vi "MAIN - Car Wash.vi"() -> ()   [LabVIEW 2015, in "Car Wash.lvlib"]
uses:
  Car Wash.lvlib
  Components/State Declaration.ctl
  Components/System Trigger.ctl
  Components/System Trigger Element.ctl
  <vilib>/Utility/error.llb/DialogTypeEnum.ctl
  Components/AMC/Read Termination Message.vi
  Components/AMC/Update Message Routing Info.vi
  Components/AMC/Create Multiple Messages.vi
  Components/AMC/Create Single Message.vi
  Components/AMC/Globals.vi
  Components/AMC/Send Message.vi
  Components/TypeDef - SHIFTER.ctl
  Components/Dependencies.llb/TLB`_Dependencies.lvlib
  Components/AMC/AMC.lvlib
panel:
  out "Status":string
  in  "Start Wash":bool
  in  "Reset Car":bool
  out "Wash Progress":i32(slide) scale=0.0..6.0
  in  "Giant Blowdryers":bool
  in  "Rinse":bool
  in  "Wax":bool
  in  "Roller Brushes":bool
  in  "Soap":bool
  in  "Pre-Soak":bool
  out "error out":errorcluster
  # "Car Wash"
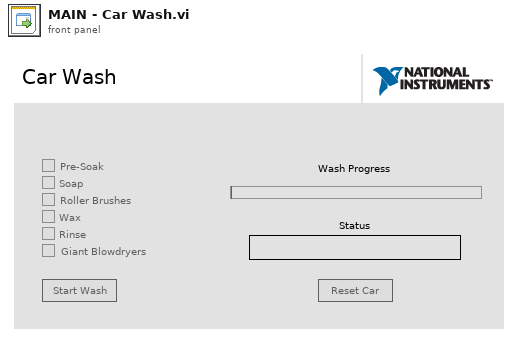
[diagram p1: front panel]
types:
  T1 = typedef "Car Wash.lvlib/System Trigger.ctl" = enum16{"<None>", "Cache User Parameters", "Close Application", "Start Wash", "Reset Car"}
  T2 = typedef "Car Wash.lvlib/State Declaration.ctl" = enum16{"<Startup>", "Idle", "Washing", "<Shutdown>"}
  T3 = enum16{"Clear SR", "Set Display", "Set Shifter", "Initialize Events", "Init Q"}
  T4 = typedef "Car Wash.lvlib/TypeDef - SHIFTER.ctl" = cluster{"State":T2, "User Data":cluster{"Active Item Tag":string, "Pre-Soak":bool, "Soap":bool, "Roller Brushes":bool, "Wax":bool, "Rinse":bool, "Giant Blowdryers":bool}, "Display Data":cluster{"Active Item Tag":string, "Wash Progress":i32, "Status":string}, "User Parameter Controls":refnum<vi>[], "Framework Data":cluster{"Exit Event":T5, "Terminate Error":errorcluster}, "Private Data":cluster{"Active Item Tag":string, "Step Booleans Array":bool[], "Step Names Array":string[], "Wash Done?":bool, "Step Duration":i32}}
  T5 = typedef "Car Wash.lvlib/TLB`_Dependencies.lvlib/Exit Event Ref.ctl" = refnum<user-event>
  T6 = typedef "Car Wash.lvlib/System Trigger Element.ctl" = cluster{"System Triggers":T1, "Trigger Data":variant}
  T7 = typedef "Car Wash.lvlib/AMC.lvlib/Message Queue.ctl" = refnum<queue>
  T8 = enum8{"Enabled", "Disabled", "Disabled and Grayed Out"}
  T9 = typedef "DialogTypeEnum.ctl" = enum16{"no dialog", "OK message", "continue or stop message", "auto error handling dialog", "OK message + warnings", "continue/stop + warnings"}
  T10 = enum32{"Invalid", "Standard", "Closed", "Hidden", "Minimized", "Maximized"}
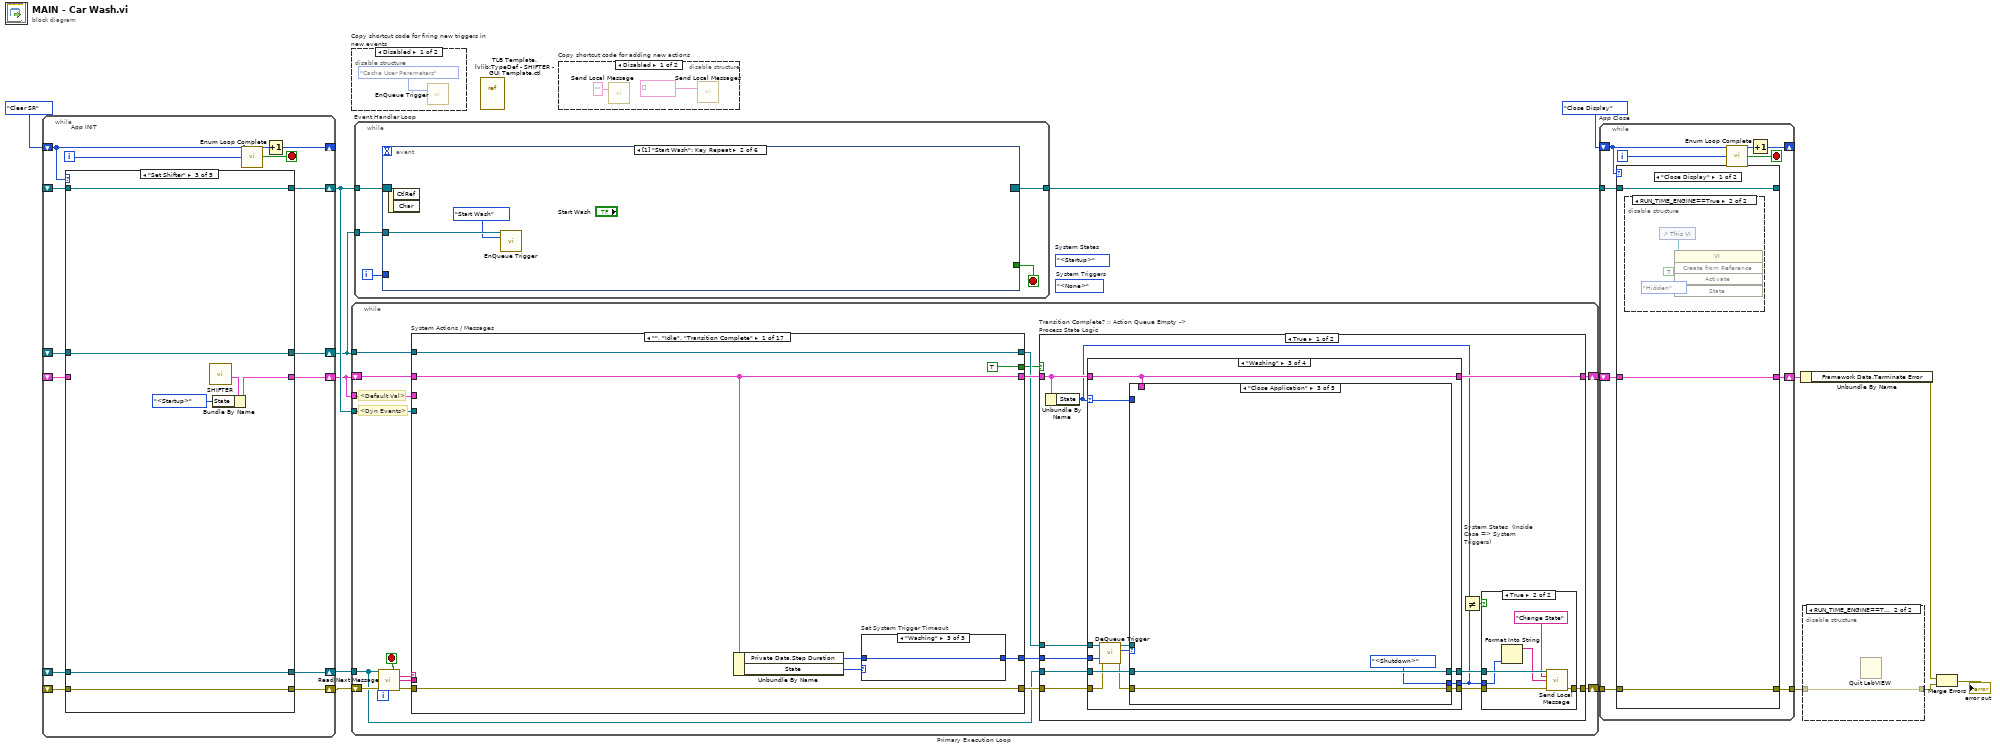
[diagram p0: block diagram]
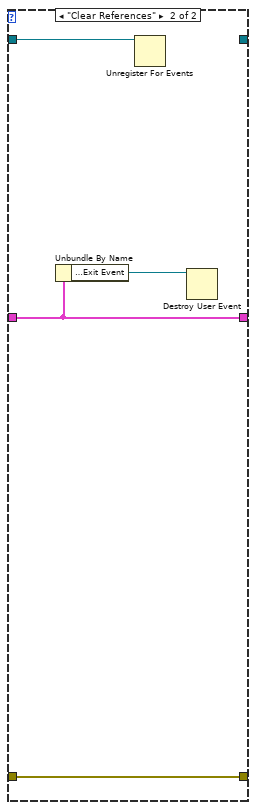
[diagram p6: hidden frame]
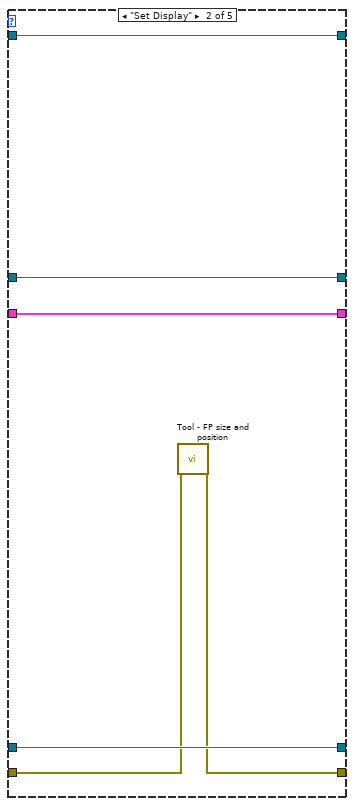
[diagram p8: hidden frame]
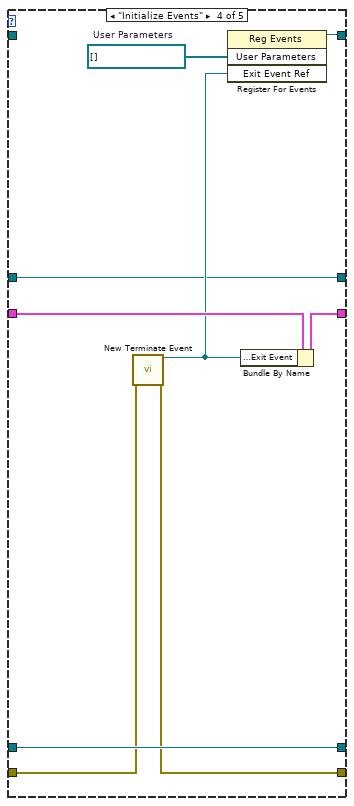
[diagram p9: hidden frame]
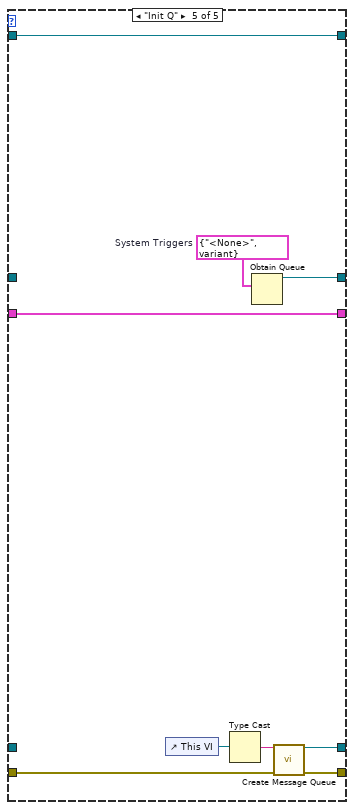
[diagram p10: hidden frame]
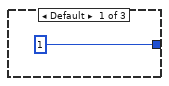
[diagram p11: hidden frame]
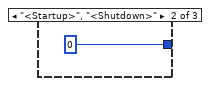
[diagram p12: hidden frame]
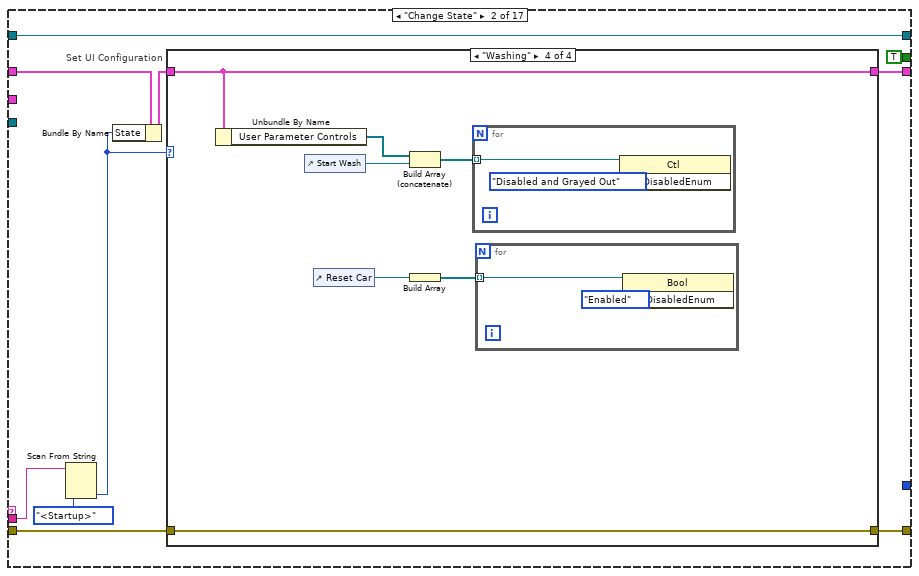
[diagram p13: hidden frame]
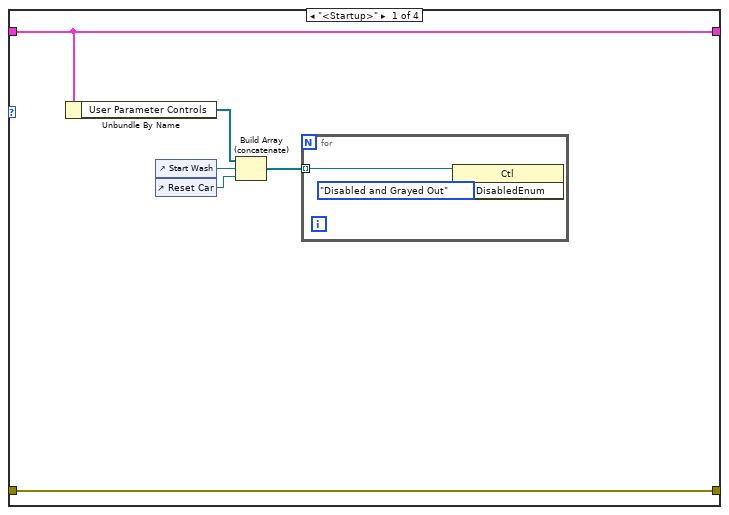
[diagram p14: hidden frame]
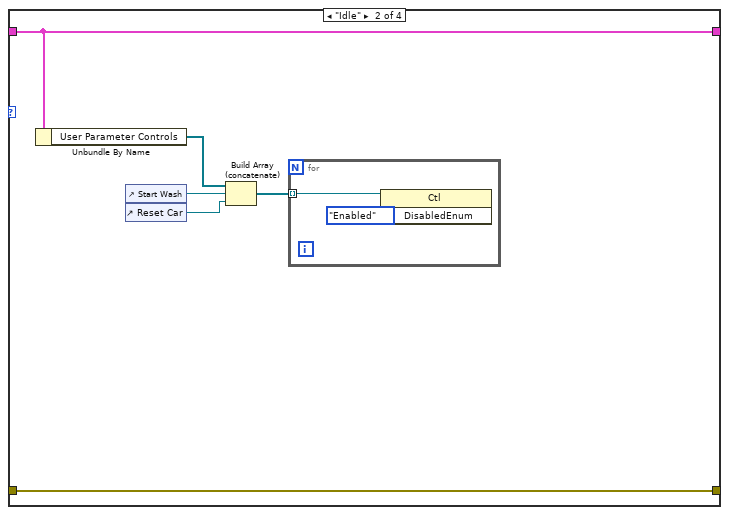
[diagram p15: hidden frame]
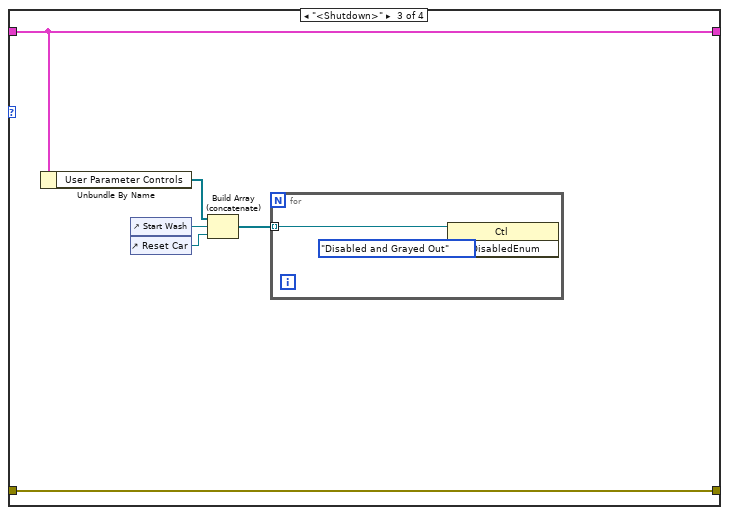
[diagram p16: hidden frame]
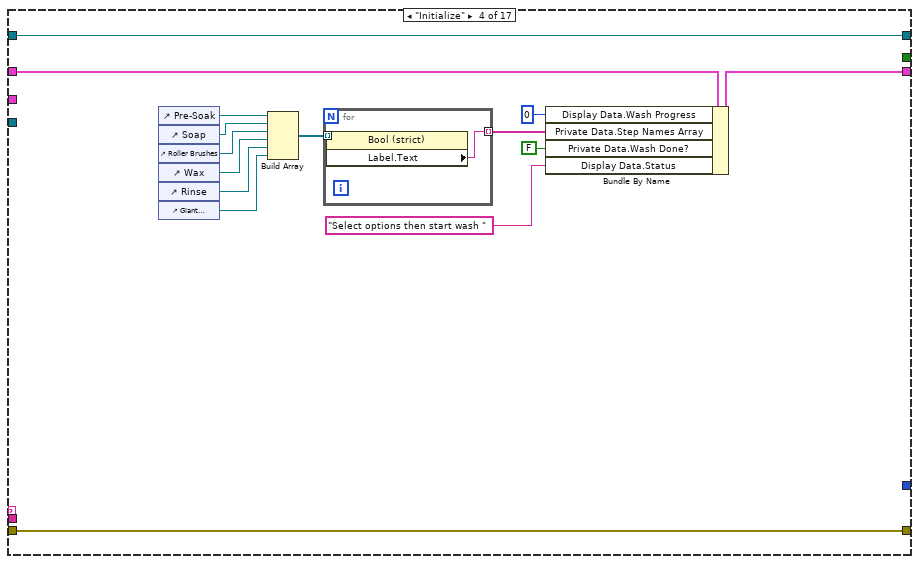
[diagram p18: hidden frame]
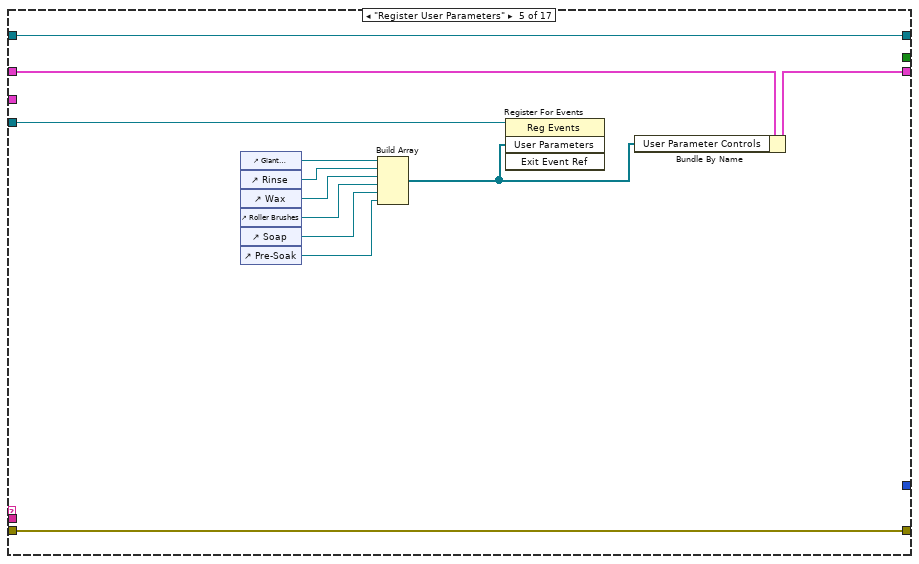
[diagram p19: hidden frame]
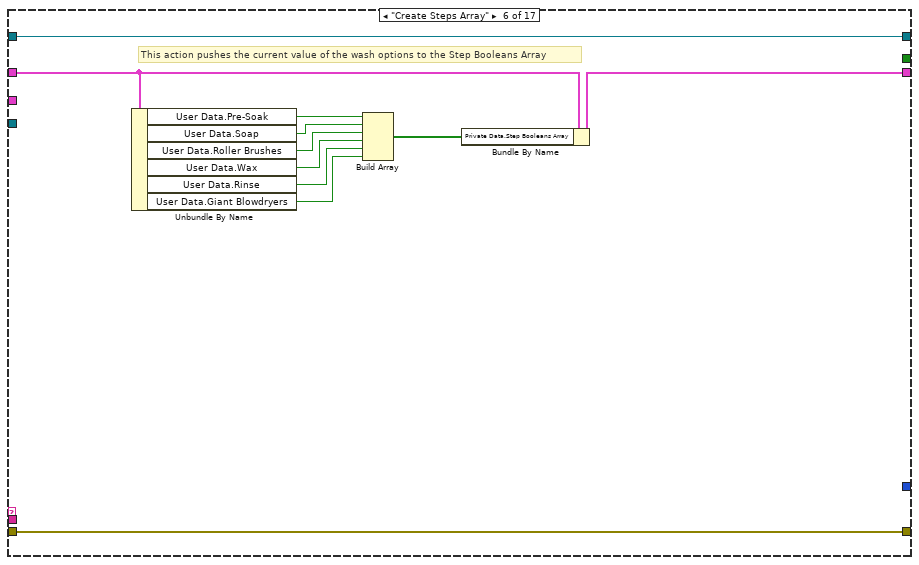
[diagram p20: hidden frame]
diagram:
  (unwired) System_Trigger."<None>"  # System Triggers
  (unwired) State_Declaration."<Startup>"  # System States
  n1 = while "App INIT" {
    shift-right: [w23] -> _
    shift-left: T3."Clear SR" -> [w18]
    shift-right: [w29] -> w9
    shift-left: _ -> [w22]
    shift-right: [w26] -> w8
    shift-left: _ -> [w21]
    shift-right: [w28] -> w11
    shift-left: _ -> [w20]
    shift-right: [w27] -> w1
    shift-left: _ -> [w19]
    shift-right: [w17] -> w2
    shift-left: _ -> [w16]
    i -> [w24]
    stop <- w25 stop-if-true
    n2 = case shown="\"Set Shifter\"" w18 {
      tunnel: [_ w33 w42 w51 w56] -> w29
      tunnel: [_ w31 w41 w44 w55] -> w26
      tunnel: [_ w35 w36 w48 w54] -> w27
      tunnel: [_ w34 w40 w47 w60] -> w28
      tunnel: w22 -> [_ w33 w42 w51 _]
      tunnel: w21 -> [_ w32 w41 w45 w59]
      tunnel: w20 -> [_ w34 w40 _ w60]
      tunnel: w19 -> [_ w35 _ w49 w54]
      tunnel: [_ w30 w39 w43 w58] -> w17
      tunnel: w16 -> [_ w30 w39 w43 _]
      frame "Clear SR" {
      }
      frame "Set Display" {
        n3 = call "Tool - FP size and position.vi"("error in (no error)"=w32) -> ("error out"=w31:errorcluster)  [unwired: 7 in, 11 out]
      }
      frame "Set Shifter" {
        n4 = call "SHIFTER.vi"() -> ("SHIFTER DATA"=w37:T4)  [unwired: 15 in]
        n5 = Bundle By Name(cluster=w37, "State"=State_Declaration."<Startup>") -> (w36:T4)
      }
      frame "Initialize Events" {
        w50 = refnum<vi>[] []  # User Parameters
        n6 = call "New Terminate Event.vi"("error in (no error)"=w45) -> ("Exit Event Ref"=w46:T5, "error out"=w44:errorcluster)  [unwired: 13 in]
        n7 = register-events(w50, w46) -> (reference out=w47:refnum<event-registration>)  [unwired: 2 in, 1 out]
        n8 = Bundle By Name(cluster=w49, "Framework Data.Exit Event"=w46) -> (w48:T4)
      }
      frame "Init Q" {
        w57 = T6 {"System Triggers"=enum."<None>", "Trigger Data"=variant}  # System Triggers
        n9 = control-ref of="This VI"() -> (w53:refnum<vi>)
        n10 = Type Cast(x=w53) -> (*(type *) &x=w52:string)  [unwired: 1 in]
        n11 = Obtain Queue(element data type=w57) -> (queue out=w58:refnum<queue>)  [unwired: 4 in, 2 out]
        n12 = call "Create Message Queue.vi"("message queue name"=w52, "error in"=w59) -> ("message queue out"=w56:T7, "error out"=w55:errorcluster)  [unwired: 12 in]
      }
    }
    n13 = call "Enum Loop Complete.vi"("Current State Enum"=w18, "Itteration"=w24) -> ("Loop Complete?"=w25:bool)  [unwired: 13 out]
    n14 = Increment(x=w18) -> (x+1=w23:T3)
  }
  n15 = disable-structure "Copy shortcut code for firing new triggers in new events" shown="Disabled" {
    frame Disabled {
      n16 = call "EnQueue Trigger.vi"("System Triggers"=System_Trigger."Cache User Parameters") -> ()  [unwired: 13 in, 2 out]
    }
    frame Enabled {
    }
  }
  n17 = while "Primary Execution Loop" {
    shift-right: [w68] -> w15
    shift-left: w8 -> [w75]
    shift-right: [w71] -> w14
    shift-left: w1 -> [w78]
    tunnel: w1 -> [w77]
    tunnel: w9 -> [w66]
    tunnel: w11 -> [w76]
    tunnel: w2 -> [w67]
    stop <- w73 stop-if-true
    # "<Dyn Events>"
    # "<Default Val>"
    n18 = call "Read Next Message.vi"("message queue in"=w66, "error in"=w75) -> ("exit process?"=w73:bool, "message name"=w72:string, "message value"=w63:string, "error out"=w74:errorcluster)  [unwired: 6 in, 4 out]
    n19 = case "System Actions / Messages" shown="\"\", \"Idle\", \"Transition Complete\"" w72 {
      selector: w72 -> [_ _ _ _ _ _ _ _ _ _ _ _ _ _ _ _ w266]
      tunnel: [w80 w93 w136 w150 w165 w176 w179 w187 w194 w197 w208 w225 w229 w232 w237 w260 w270] -> w69
      tunnel: w74 -> [w80 w92 w136 w150 w165 w176 w179 w187 w194 w197 w208 w225 w229 w232 w238 w259 w271]
      tunnel: w78 -> [w81 w89 w135 w146 w164 w169 w178 w189 w192 w195 w201 w221 w227 w231 w235 w263 w272]
      tunnel: w77 -> [_ _ _ _ _ _ _ _ _ _ _ _ _ _ _ _ _]
      tunnel: [w81 w91 w135 w149 w163 w168 w178 w188 w192 w195 w200 w223 w227 w231 w236 w263 w272] -> w70
      tunnel: [w82 _ _ _ _ _ _ _ _ _ _ _ w226 _ _ _ _] -> w62
      tunnel: w76 -> [_ _ _ _ w162 _ _ _ _ _ _ _ _ _ _ _ _]
      tunnel: [w84 w97 w134 w151 w161 w175 w177 w186 w193 w196 w207 w224 w228 w230 w233 w257 w264] -> w65
      tunnel: w67 -> [w84 w97 w134 w151 w161 w175 w177 w186 w193 w196 w207 w224 w228 w230 w233 w257 w264]
      tunnel: [TRUE TRUE _ _ _ _ _ _ _ _ _ _ _ _ _ _ _] -> w64
      tunnel: w63 -> [_ w96 _ _ _ _ _ _ _ _ _ _ _ _ _ _ _]
      frame "", "Idle", "Transition Complete" {
        n20 = Unbundle By Name(w81) -> ("Private Data.Step Duration"=w79:i32, "State"=w83:T2)
        n21 = case "Set System Trigger Timeout" shown="\"Washing\"" w83 {
          tunnel: [1 0 w88] -> w82
          tunnel: w79 -> [_ _ w88]
          frame Default {
          }
          frame "<Startup>", "<Shutdown>" {
          }
          frame "Washing" {
          }
        }
      }
      frame "Change State" {
        n22 = Scan From String(input string=w96, default 1=State_Declaration."<Startup>" ("State")) -> (output 1=w94:T2)  [unwired: 3 in, 3 out]
        n23 = Bundle By Name(cluster=w89, "State"=w94) -> (w90:T4)
        n24 = case "Set UI Configuration" shown="\"Washing\"" w94 {
          tunnel: [w104 w112 w120 w129] -> w93
          tunnel: w92 -> [w104 w112 w120 w129]
          tunnel: [w100 w108 w116 w124] -> w91
          tunnel: w90 -> [w100 w108 w116 w124]
          frame "<Startup>" {
            n25 = Unbundle By Name(w100) -> ("User Parameter Controls"=w99:refnum<vi>[])
            n26 = control-ref of="Start Wash"() -> (w103:refnum<vi>)
            n27 = control-ref of="Reset Car"() -> (w101:refnum<vi>)
            n28 = Build Array (concatenate)(w99, w103, w101) -> (w102:refnum<vi>[])
            n29 = for {
              tunnel: w102 -> [w106] mode=indexing
              n30 = property class="Ctl"(reference=w106, "DisabledEnum"=T8."Disabled and Grayed Out" ("Disabled")) -> ()  [unwired: 1 in, 2 out]
            }
          }
          frame "Idle" {
            n31 = Unbundle By Name(w108) -> ("User Parameter Controls"=w107:refnum<vi>[])
            n32 = control-ref of="Start Wash"() -> (w110:refnum<vi>)
            n33 = control-ref of="Reset Car"() -> (w109:refnum<vi>)
            n34 = Build Array (concatenate)(w107, w110, w109) -> (w111:refnum<vi>[])
            n35 = for {
              tunnel: w111 -> [w114] mode=indexing
              n36 = property class="Ctl"(reference=w114, "DisabledEnum"=T8."Enabled" ("Disabled")) -> ()  [unwired: 1 in, 2 out]
            }
          }
          frame "<Shutdown>" {
            n37 = Unbundle By Name(w116) -> ("User Parameter Controls"=w115:refnum<vi>[])
            n38 = control-ref of="Start Wash"() -> (w118:refnum<vi>)
            n39 = control-ref of="Reset Car"() -> (w117:refnum<vi>)
            n40 = Build Array (concatenate)(w115, w118, w117) -> (w119:refnum<vi>[])
            n41 = for {
              tunnel: w119 -> [w122] mode=indexing
              n42 = property class="Ctl"(reference=w122, "DisabledEnum"=T8."Disabled and Grayed Out" ("Disabled")) -> ()  [unwired: 1 in, 2 out]
            }
          }
          frame "Washing" {
            n43 = Unbundle By Name(w124) -> ("User Parameter Controls"=w123:refnum<vi>[])
            n44 = control-ref of="Start Wash"() -> (w127:refnum<vi>)
            n45 = control-ref of="Reset Car"() -> (w125:refnum<vi>)
            n46 = Build Array (concatenate)(w123, w127) -> (w128:refnum<vi>[])
            n47 = Build Array(w125) -> (w126:refnum<vi>[])
            n48 = for {
              tunnel: w128 -> [w133] mode=indexing
              n49 = property class="Ctl"(reference=w133, "DisabledEnum"=T8."Disabled and Grayed Out" ("Disabled")) -> ()  [unwired: 1 in, 2 out]
            }
            n50 = for {
              tunnel: w126 -> [w131] mode=indexing
              n51 = property class="Bool"(reference=w131, "DisabledEnum"=T8."Enabled" ("Disabled")) -> ()  [unwired: 1 in, 2 out]
            }
          }
        }
      }
      frame "/*********Initialize********/" {
      }
      frame "Initialize" {
        n52 = control-ref of="Pre-Soak"() -> (w143:refnum<vi>)
        n53 = control-ref of="Soap"() -> (w142:refnum<vi>)
        n54 = control-ref of="Roller Brushes"() -> (w141:refnum<vi>)
        n55 = control-ref of="Wax"() -> (w140:refnum<vi>)
        n56 = control-ref of="Rinse"() -> (w139:refnum<vi>)
        n57 = control-ref of="Giant Blowdryers"() -> (w138:refnum<vi>)
        n58 = Build Array(w143, w142, w141, w140, w139, w138) -> (w144:refnum<vi>[])
        n59 = for {
          tunnel: w144 -> [w152] mode=indexing
          tunnel: [w153] -> w145 mode=indexing
          n60 = property class="Bool (strict)"(reference=w152) -> ("Label.Text"=w153:string)  [unwired: 1 in, 2 out]
        }
        n61 = Bundle By Name(cluster=w146, "Display Data.Wash Progress"=0, "Private Data.Step Names Array"=w145, "Private Data.Wash Done?"=FALSE, "Display Data.Status"="Select options then start wash " ("Status")) -> (w149:T4)
      }
      frame "Register User Parameters" {
        n62 = control-ref of="Giant Blowdryers"() -> (w160:refnum<vi>)
        n63 = control-ref of="Rinse"() -> (w155:refnum<vi>)
        n64 = control-ref of="Wax"() -> (w156:refnum<vi>)
        n65 = control-ref of="Roller Brushes"() -> (w157:refnum<vi>)
        n66 = control-ref of="Soap"() -> (w158:refnum<vi>)
        n67 = control-ref of="Pre-Soak"() -> (w159:refnum<vi>)
        n68 = Build Array(w160, w155, w156, w157, w158, w159) -> (w154:refnum<vi>[])
        n69 = register-events(reference=w162, w154) -> ()  [unwired: 2 in, 2 out]
        n70 = Bundle By Name(cluster=w164, "User Parameter Controls"=w154) -> (w163:T4)
      }
      frame "Create Steps Array" {
        # "This action pushes the current value of the wash options to the Step Booleans Array"
        n71 = Unbundle By Name(w169) -> ("User Data.Pre-Soak"=w166:bool, "User Data.Soap"=w174:bool, "User Data.Roller Brushes"=w173:bool, "User Data.Wax"=w172:bool, "User Data.Rinse"=w171:bool, "User Data.Giant Blowdryers"=w170:bool)
        n72 = Build Array(w166, w174, w173, w172, w171, w170) -> (w167:bool[])
        n73 = Bundle By Name(cluster=w169, "Private Data.Step Booleans Array"=w167) -> (w168:T4)
      }
      frame "/*********Display Updates********/" {
      }
      frame "Cache User Parameters" {
        # "This Action reads the control values and places the data into the Mother Cluster"
        n74 = Bundle By Name(cluster=w189, "User Data.Pre-Soak"="Pre-Soak", "User Data.Soap"="Soap", "User Data.Roller Brushes"="Roller Brushes", "User Data.Wax"="Wax", "User Data.Rinse"="Rinse", "User Data.Giant Blowdryers"="Giant Blowdryers") -> (w188:T4)
      }
      frame "Update Display" {
        n75 = Unbundle By Name(w192) -> ("Display Data.Wash Progress"=→"Wash Progress":i32, "Display Data.Status"=→"Status":string)
      }
      frame "/*********Primary Execution********/" {
      }
      frame "Evaluate Step" {
        n76 = Unbundle By Name(w201) -> ("Display Data.Wash Progress"=w204:i32, "Private Data.Step Booleans Array"=w206:bool[], "Private Data.Step Names Array"=w205:string[])
        n77 = Index Array(array=w205, index=w204) -> (element=w203:string)
        n78 = Index Array(array=w206, index=w204) -> (element=w202:bool)
        n79 = case shown="False" w202 {
          tunnel: w203 -> [_ w212]
          tunnel: ["" ("String") w212] -> w199
          tunnel: [0 ("Private Data.Step Duration") 1000 ("Private Data.Step Duration")] -> w198
          frame False {
            # "Do nothing\ndo not execute the wash option\ndo not update the status"
          }
          frame True {
          }
        }
        n80 = Bundle By Name(cluster=w201, "Private Data.Step Duration"=w198, "Display Data.Status"=w199) -> (w200:T4)
      }
      frame "Increment Step" {
        # "increment the Wash Progress value\nCheck if the washing cycle is complete"
        n81 = Unbundle By Name(w221) -> ("Display Data.Wash Progress"=w219:i32, "Private Data.Step Booleans Array"=w220:bool[], "Display Data.Status"=w213:string)
        n82 = Array Size(array=w220) -> (size(s)=w222:i32)
        n83 = Increment(x=w219) -> (x+1=w218:i32)
        n84 = Decrement(x=w222) -> (x-1=w217:i32)
        n85 = Greater Or Equal?(x=w218, y=w217) -> (x >= y?=w215:bool)
        n86 = Select(t="Washing Complete", s=w215, f=w213) -> (s? t:f=w214:string)
        n87 = Bundle By Name(cluster=w221, "Display Data.Wash Progress"=w218, "Private Data.Wash Done?"=w215, "Display Data.Status"=w214) -> (w223:T4)
      }
      frame "Set Step Duration" {
        # "This action needs to be called last so that\nthe timeout is triggered. A timeout is triggered\nafter x ms without a system trigger."
        n88 = Unbundle By Name(w227) -> ("Private Data.Step Duration"=w226:i32)
      }
      frame "/*********Shutdown********/" {
      }
      frame "Error" {
        n89 = Unbundle By Name(w235) -> ("State"=w234:T2)
        n90 = case shown="Default" w234 {
          tunnel: w238 -> [w246]
          tunnel: [w245] -> w237
          tunnel: w235 -> [w242]
          tunnel: [w241] -> w236
          tunnel: w233 -> [w239]
          frame Default {
            n91 = call <vilib>:"General Error Handler CORE.vi"("type of dialog (OK msg:1)"=DialogTypeEnum."auto error handling dialog", "error in (no error)"=w246) -> ("stop event propagated"=w244:bool, "error out"=w240:errorcluster)  [unwired: 12 out]
            n92 = case "User Chose to Stop and Not Continue\nFALSE = Continue: CLEAR ERRORS" shown="False" w244 {
              tunnel: [w247 w252] -> w245
              tunnel: w240 -> [w248 w254]
              tunnel: w242 -> [w249 w256]
              tunnel: [w249 w255] -> w241
              tunnel: w239 -> [_ w253]
              frame False {
                n93 = call <vilib>:"Clear Errors.vi"("error in (no error)"=w248) -> ("error out"=w247:errorcluster)  [unwired: 1 in, 5 out]
              }
              frame True {
                n94 = call <vilib>:"Clear Errors.vi"("error in (no error)"=w254) -> ("error out"=w251:errorcluster)  [unwired: 1 in, 5 out]
                n95 = Bundle By Name(cluster=w256, "Framework Data.Terminate Error"=w254) -> (w255:T4)
                n96 = call "EnQueue Trigger.vi"("Queue in"=w253, "System Triggers"=System_Trigger."Close Application", "error in (no error)"=w251) -> ("error out"=w252:errorcluster)  [unwired: 11 in, 1 out]
              }
            }
          }
        }
      }
      frame "Exit" {
        w258 = refnum<class> refnum  # event data
        # "Don't wire 'Error In'\nMust Execute Regardless"
        n97 = Unbundle By Name(w263) -> ("Framework Data.Exit Event"=w262:T5)  [unwired: 1 out]
        n98 = Generate User Event(user event=w262, event data cluster=w258) -> (error out=w261:errorcluster)  [unwired: 2 in, 1 out]
        n99 = Merge Errors(w261, w259) -> (w260:errorcluster)
      }
      frame Default {
        w268 = 1 items=["No error", "Argument error", "Memory is full", "Out of zone", "End of file", "File already open", "Generic file I/O error", "File not found", "File permission error", "Disk is full", "Duplicate path", "Too many files open", "System feature not enabled", "Resource file not found", "Cannot add resource", "Resource not found", "Image not found", "Image memory error", "Pen does not exist", "Config type invalid", "Config token not found", "Config parse error", "Config memory error", "Bad external code format", "Bad external code offset", "External code not present", "Null window", "Destroy window error", "Null menu", "Print aborted", "Bad print record", "Print driver error", "Windows error during printing", "Memory error during printing", "Print dialog error", "Generic print error", "Invalid device refnum", "Device not found", "Device parameter error", "Device unit error", "Cannot open device", "Device call aborted", "Generic error", "Cancelled by user", "Object ID too low", "Object ID too high", "Object not in heap", "Unknown heap", "Unknown object (invalid DefProc)", "Unknown object (DefProc not in table)", "Message out of range", "Invalid (null) method", "Unknown message", "Manager call not supported", "Bad address", "Network operation in progress", "Network operation timed out", "Connection is busy", "Network attribute not supported", "Network error", "Address in use", "System out of memory", "Connection aborted", "Connection refused", "Not connected", "Already connected", "Connection closed", "Initialization error (interapplication manager)", "Bad occurrence", "Wait on unbound occurrence handler", "Occurrence queue overflow", "Datalog type conflict", "Unused", "Unrecognized type (interapplication manager)", "Memory corrupt", "Failed to make temporary DLL", "Old CIN version", "Drag socket not found", "Failed to load drop-object", "Failed to register OLE object", "Failed to release OLE object", "Format specifier type mismatch", "Unknown format specifier", "Too few format specifiers", "Too many format specifiers", "Scan failed", "Newer CIN version", "Error converting to variant", "Runtime menu error", "Password tampered", "Variant attribute not found", "Incompatible variant data type", "Event data is not available", "Event Store is not present", "Occurrence is not found", "Event Queue is not created", "Event info is not available", "Refnum passed is NULL", "Error retrieving Class GUID", "Error retrieving CoClass GUID", "Error retrieving TypeLib GUID.", "Bad built application magic bytes.", "Specific driver is different from the specific driver associated with the Logical Name.", "There is no session opened to the class driver.", "Max Error", "MAX - Error with config objects", "MAX - Error loading configuration", "MAX - Group not supported"]
        w269 = TRUE  # status
        n100 = Format Into String(format string="DEVELOPER ERROR:\nImproper Action Requested\n================\nAction {%s} does not exist within this architecture\n\nCheck for spelling and case errors" ("source"), w266) -> (resulting string=w267:string)  [unwired: 2 in, 1 out]
        n101 = Bundle By Name(cluster=w271, "status"=w269, "code"=w268, "source"=w267) -> (w270:errorcluster)
      }
    }
    n102 = case "Transition Complete? :: Action Queue Empty -> Process State Logic" shown="True" w64 {
      tunnel: [w284 w406] -> w71
      tunnel: w70 -> [w274 w406]
      tunnel: w69 -> [w283 w405]
      tunnel: w66 -> [w282 _]
      tunnel: [w278 w405] -> w68
      tunnel: w65 -> [w281 _]
      tunnel: w62 -> [w275 _]
      frame True {
        n103 = Unbundle By Name(w274) -> ("State"=w273:T2)
        n104 = case "System States  (Inside Case => System Triggers)" shown="\"Washing\"" w273 {
          selector: w273 -> [_ w313 w353 _]
          tunnel: [w300 w319 w348 w396] -> w284
          tunnel: w274 -> [w300 w319 w348 w396]
          tunnel: w283 -> [w294 w311 w351 w390]
          tunnel: w282 -> [w292 w315 w355 w388]
          tunnel: [w299 w318 w358 w395] -> w279
          tunnel: w281 -> [w302 w320 w359 w398]
          tunnel: [w298 w317 w357 w394] -> w280
          tunnel: [w297 w316 w356 w393] -> w277
          tunnel: w275 -> [w296 w309 w349 w392]
          frame "<Startup>" {
            n105 = call "DeQueue Trigger.vi"("Queue in"=w302, "Timeout (0)"=w296, "error in (no error)"=w294) -> ("Queue out"=w295:refnum<queue>, "System Triggers"=w301:T1, "error out"=w293:errorcluster)  [unwired: 9 in, 1 out]
            n106 = case shown="\"<None>\", Default" w301 {
              tunnel: w300 -> [_]
              tunnel: [w306] -> w299
              tunnel: w293 -> [w307]
              tunnel: w292 -> [w305]
              tunnel: [w304] -> w298
              tunnel: [State_Declaration."Idle" ("State")] -> w297
              tunnel: w295 -> [_]
              frame "<None>", Default {
                w303 = string[] ["Initialize", "Cache User Parameters", "Register User Parameters", "Update Display"]  # Initial Elements
                n107 = call "Send Local Messages.vi"("message queue in"=w305, "message names"=w303, "error in"=w307) -> ("message queue out"=w304:T7, "error out"=w306:errorcluster)  [unwired: 10 in, 1 out]
              }
            }
          }
          frame "Idle" {
            n108 = call "DeQueue Trigger.vi"("Queue in"=w320, "Timeout (0)"=w309, "error in (no error)"=w311) -> ("Queue out"=w314:refnum<queue>, "System Triggers"=w312:T1, "error out"=w310:errorcluster)  [unwired: 9 in, 1 out]
            n109 = case shown="\"Start Wash\"" w312 {
              tunnel: w319 -> [_ _ _ _ _ _]
              tunnel: [w321 w325 w329 w334 w336 w342] -> w318
              tunnel: w310 -> [w321 w325 w332 w334 w339 w345]
              tunnel: w315 -> [w322 w326 w331 w335 w337 w343]
              tunnel: [w322 w326 w330 w335 w338 w344] -> w317
              tunnel: [State_Declaration."Idle" ("State") State_Declaration."<Shutdown>" ("State") w327 State_Declaration."Idle" ("State") State_Declaration."Washing" ("State") State_Declaration."Idle" ("State")] -> w316
              tunnel: w314 -> [_ _ _ _ _ _]
              tunnel: w313 -> [_ _ w327 _ _ _]
              frame "<None>" {
              }
              frame "Close Application" {
              }
              frame "Cache User Parameters" {
                n110 = call "Send Local Message.vi"("message queue in"=w331, "message name"="Cache User Parameters" ("Message Name"), "error in"=w332) -> ("message queue out"=w330:T7, "error out"=w329:errorcluster)  [unwired: 10 in, 1 out]
              }
              frame Default {
              }
              frame "Start Wash" {
                # "next state to go to"
                # "Actions to perform"
                n111 = call "Send Local Messages.vi"("message queue in"=w337, "message names"=string[] ["Initialize", "Update Display", "Create Steps Array"], "error in"=w339) -> ("message queue out"=w338:T7, "error out"=w336:errorcluster)  [unwired: 10 in, 1 out]
              }
              frame "Reset Car" {
                # "Next State"
                # "Actions to perform"
                n112 = call "Send Local Messages.vi"("message queue in"=w343, "message names"=string[] ["Initialize", "Update Display"], "error in"=w345) -> ("message queue out"=w344:T7, "error out"=w342:errorcluster)  [unwired: 10 in, 1 out]
              }
            }
          }
          frame "Washing" {
            n113 = call "DeQueue Trigger.vi"("Queue in"=w359, "Timeout (0)"=w349, "error in (no error)"=w351) -> ("Queue out"=w354:refnum<queue>, "System Triggers"=w352:T1, "error out"=w350:errorcluster)  [unwired: 9 in, 1 out]
            n114 = case shown="\"Close Application\"" w352 {
              tunnel: w348 -> [w365 _ _ _ _]
              tunnel: [w368 w374 w377 w381 w386] -> w358
              tunnel: w350 -> [w369 w375 w377 w384 w386]
              tunnel: w355 -> [w367 w373 w378 w383 w387]
              tunnel: [w366 w372 w378 w382 w387] -> w357
              tunnel: [w362 State_Declaration."Idle" ("State") State_Declaration."<Shutdown>" ("State") w379 State_Declaration."Washing" ("State")] -> w356
              tunnel: w354 -> [_ _ _ _ _]
              tunnel: w353 -> [_ _ _ w379 _]
              frame "<None>" {
                # "Conditional next state"
                # "action list"
                n115 = Unbundle By Name(w365) -> ("Private Data.Wash Done?"=w361:bool)
                n116 = call "Send Local Messages.vi"("message queue in"=w367, "message names"=string[] ["Evaluate Step", "Increment Step", "Update Display"], "error in"=w369) -> ("message queue out"=w366:T7, "error out"=w368:errorcluster)  [unwired: 10 in, 1 out]
                n117 = Select(t=State_Declaration."Idle" ("State"), s=w361, f=State_Declaration."Washing" ("State")) -> (s? t:f=w362:T2)
              }
              frame "Reset Car" {
                n118 = call "Send Local Messages.vi"("message queue in"=w373, "message names"=string[] ["Initialize", "Update Display"], "error in"=w375) -> ("message queue out"=w372:T7, "error out"=w374:errorcluster)  [unwired: 10 in, 1 out]
              }
              frame "Close Application" {
              }
              frame "Cache User Parameters" {
                n119 = call "Send Local Message.vi"("message queue in"=w383, "message name"="Cache User Parameters" ("Message Name"), "error in"=w384) -> ("message queue out"=w382:T7, "error out"=w381:errorcluster)  [unwired: 10 in, 1 out]
              }
              frame Default {
              }
            }
          }
          frame "<Shutdown>" {
            n120 = call "DeQueue Trigger.vi"("Queue in"=w398, "Timeout (0)"=w392, "error in (no error)"=w390) -> ("Queue out"=w391:refnum<queue>, "System Triggers"=w397:T1, "error out"=w389:errorcluster)  [unwired: 9 in, 1 out]
            n121 = case shown="\"<None>\", Default" w397 {
              tunnel: w396 -> [_]
              tunnel: [w399] -> w395
              tunnel: w389 -> [w401]
              tunnel: w388 -> [w402]
              tunnel: [w400] -> w394
              tunnel: [State_Declaration."<Shutdown>" ("State")] -> w393
              tunnel: w391 -> [_]
              frame "<None>", Default {
                n122 = call "Send Local Messages.vi"("message queue in"=w402, "message names"=string[] ["Exit"], "error in"=w401) -> ("message queue out"=w400:T7, "error out"=w399:errorcluster)  [unwired: 10 in, 1 out]
              }
            }
          }
        }
        n123 = Not Equal?(x=w273, y=w277) -> (x != y?=w276:bool)
        n124 = case shown="True" w276 {
          tunnel: w280 -> [_ w291]
          tunnel: w279 -> [w285 w290]
          tunnel: [w285 w289] -> w278
          tunnel: w277 -> [_ w287]
          frame False {
          }
          frame True {
            n125 = Format Into String(w287) -> (resulting string=w286:string)  [unwired: 3 in, 1 out]
            n126 = call "Send Local Message.vi"("message queue in"=w291, "message name"="Change State" ("Message Name"), "message value"=w286, "error in"=w290) -> ("error out"=w289:errorcluster)  [unwired: 9 in, 2 out]
          }
        }
      }
      frame False {
      }
    }
  }
  n127 = while "Event Handler Loop" {
    tunnel: w11 -> [w410]
    tunnel: [w409] -> w13
    tunnel: w2 -> [w407]
    i -> [w408]
    stop <- w411 stop-if-true
    n128 = event shown="[1] \"Start Wash\": Key Repeat" {
      selector: w410 -> [_ _ _ _ _ _]
      dyn-events: [_ _ _ _ _ _] -> w409
      timeout: _ -> [_ _ _ _ _ _]
      tunnel: [_ _ _ _ TRUE ("NewVal") _] -> w411
      tunnel: w408 -> [_ _ _ _ _ _]
      tunnel: w407 -> [w413 w416 w418 _ w429 w433]
      event Panel Close? {
        w414 = TRUE  # Discard?
        n129 = event-data() -> ()  [unwired: 2 out]
        n130 = call "EnQueue Trigger.vi"("Queue in"=w413, "System Triggers"=System_Trigger."Close Application") -> ()  [unwired: 12 in, 2 out]
        n131 = event-data("Discard?"=w414) -> ()  [unwired: 1 in, 1 out]
      }
      event "Start Wash": Value Change {
        n132 = event-data() -> ()  [unwired: 3 out]
        n133 = call "EnQueue Trigger.vi"("Queue in"=w416, "System Triggers"=System_Trigger."Start Wash") -> ()  [unwired: 12 in, 2 out]
      }
      event "Reset Car": Value Change {
        n134 = event-data() -> ()  [unwired: 3 out]
        n135 = call "EnQueue Trigger.vi"("Queue in"=w418, "System Triggers"=System_Trigger."Reset Car") -> ()  [unwired: 12 in, 2 out]
      }
      event Mouse Down {
        n136 = event-data() -> ("Param5"=w423:u16, "Param6"=w424:cluster{"Double Click":bool, "Menu Key":bool})  [unwired: 1 out]
        n137 = Unbundle By Name(w424) -> ("Double Click"=w420:bool)
        n138 = Equal?(x=u16 2, y=w423) -> (x = y?=w421:bool)
        n139 = And(x=w421, y=w420) -> (x .and. y?=w419:bool)
        n140 = case "Toggle Menu Visibility :: double RIGHT click on logo" shown="True" w419 {
          frame False {
          }
          frame True {
            n141 = property class="VI"() -> (reference out=w427:refnum<vi>, "TB.Visible"=w425:bool)  [unwired: 2 in, 1 out]
            n142 = Not(x=w425) -> (.not. x?=w426:bool)
            n143 = property class="VI"(reference=w427, "TB.Visible"=w426) -> ()  [unwired: 1 in, 2 out]
          }
        }
      }
      event User Event {
        n144 = event-data() -> ()  [unwired: 2 out]
        n145 = call "EnQueue Trigger.vi"("Queue in"=w429, "System Triggers"=System_Trigger."Close Application") -> ()  [unwired: 12 in, 2 out]
      }
      event Value Change {
        n146 = event-data() -> ()  [unwired: 2 out]
        n147 = call "EnQueue Trigger.vi"("Queue in"=w433, "System Triggers"=System_Trigger."Cache User Parameters") -> ("Queue out"=w432:refnum<queue>)  [unwired: 12 in, 1 out]
        n148 = event "use this event case to register a SPEICIFIC 'User Parameter' for a SPECIFIC action" shown="[0] Timeout" {
          selector: _ -> [_]
          dyn-events: _ -> [_]
          timeout: 0 -> [_]
          tunnel: w432 -> [_]
          event Timeout {
            n149 = event-data() -> ()  [unwired: 1 in, 1 out]
          }
        }
      }
    }
  }
  n150 = vi-ref "TLB Template.lvlib:TypeDef - SHIFTER - GUI Template.ctl"() -> ()  [unwired: 1 out]
  n151 = disable-structure "Copy shortcut code for adding new actions" shown="Disabled" {
    frame Disabled {
      n152 = call "Send Local Message.vi"("message name"="") -> ()  [unwired: 12 in, 3 out]
      n153 = call "Send Local Messages.vi"("message names"=string[] []) -> ()  [unwired: 12 in, 3 out]
    }
    frame Enabled {
    }
  }
  n154 = while "App Close" {
    shift-right: [w443] -> _
    shift-left: enum16{"Close Display", "Clear References"}."Close Display" -> [w442]
    tunnel: w13 -> [w440]
    tunnel: w15 -> [w441]
    tunnel: [w438] -> w7
    shift-right: [w437] -> w5
    shift-left: w14 -> [w439]
    i -> [w444]
    stop <- w445 stop-if-true
    n155 = case shown="\"Close Display\"" w442 {
      tunnel: [w447 w455] -> w438
      tunnel: [w446 w454] -> w437
      tunnel: [w448 _] -> _
      tunnel: w441 -> [w447 w455]
      tunnel: w440 -> [w448 w452]
      tunnel: w439 -> [w446 w454]
      frame "Close Display" {
        n156 = disable-structure shown="RUN_TIME_ENGINE==True" {
          frame condition #0 (active) {
          }
          frame condition #1 {
            n157 = control-ref of="This VI"() -> (w449:refnum<vi>)
            n158 = invoke class="VI" method="Create from Reference"(reference=w449, "Activate"=TRUE ("Activate?"), "State"=T10."Hidden") -> ()  [unwired: 2 in, 5 out]
          }
        }
      }
      frame "Clear References" {
        n159 = Unbundle By Name(w454) -> ("Framework Data.Exit Event"=w453:T5)
        n160 = Unregister For Events(event registration refnum=w452) -> ()  [unwired: 1 in, 1 out]
        n161 = Destroy User Event(user event=w453) -> ()  [unwired: 1 in, 1 out]
      }
    }
    n162 = call "Enum Loop Complete.vi"("Current State Enum"=w442, "Itteration"=w444) -> ("Loop Complete?"=w445:bool)  [unwired: 13 out]
    n163 = Increment(x=w442) -> (x+1=w443:enum16{"Close Display", "Clear References"})
  }
  n164 = Unbundle By Name(w5) -> ("Framework Data.Terminate Error"=w3:errorcluster)
  n165 = disable-structure shown="RUN_TIME_ENGINE==True" {
    disable-tunnel: [w456 w457] -> w4
    disable-tunnel: w7 -> [w456 w457]
    frame condition #0 (active) {
    }
    frame condition #1 {
      n166 = Quit LabVIEW() -> ()  [unwired: 1 in]
    }
  }
  n167 = Merge Errors(w3, w4) -> (→"error out":errorcluster)
